vi "Write File ini.vi"(8 "error in (no error)":errorcluster, 11 "ini Path":path) -> (0 "error out":errorcluster)   [LabVIEW 2015, in "Telegram Library.lvlib"]
doc: "Created IvanLis by LabVIEW Portal\nProfile: http://labviewportal.org/memberlist.php?mode=viewprofile&u=987\neMail: IvanLisanov@gMail.com\nTelegram: https://t.me/IvanLis"
uses:
  Telegram Library.lvlib
  <vilib>/Utility/config.llb/Write Key (String).vi
  <vilib>/Utility/config.llb/Write Key (Boolean).vi
  <vilib>/Utility/config.llb/Write Key (I32).vi
  <vilib>/Utility/config.llb/NI_LVConfig.lvlib
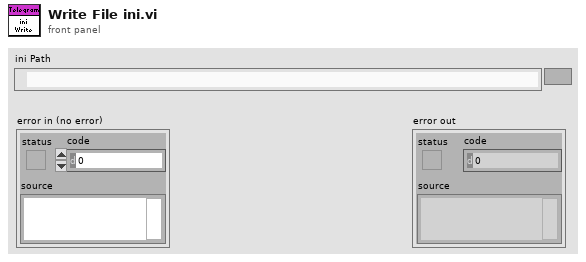
[diagram p1: front panel]
types:
  T1 = typedef "NI_LVConfig.lvlib/Config Data RefNum.ctl" = refnum<k1>
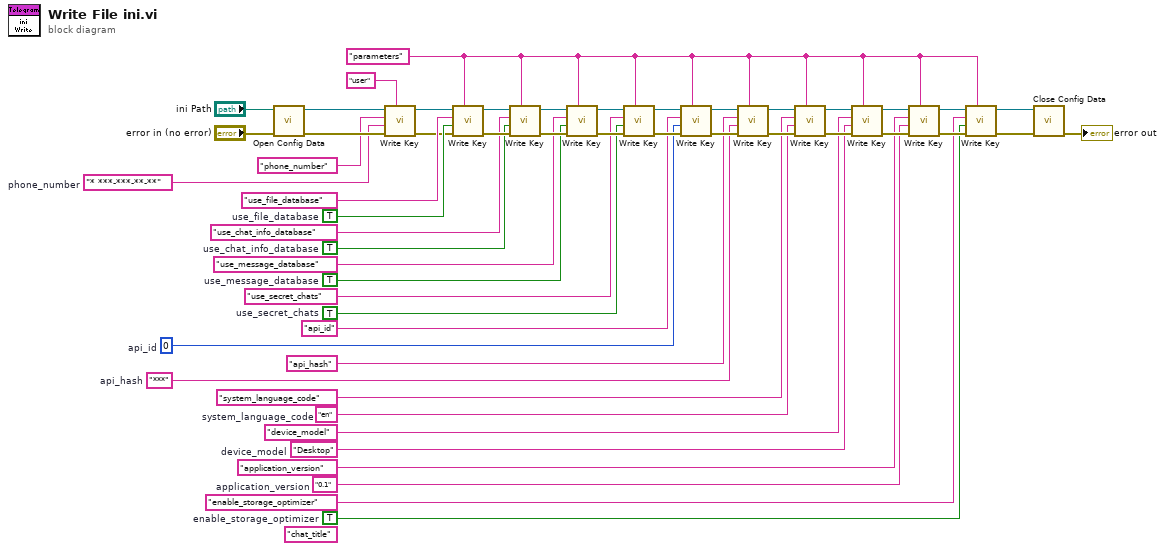
[diagram p0: block diagram]
diagram:
  w6 = TRUE  # enable_storage_optimizer
  w8 = "0.1"  # application_version
  w10 = "Desktop"  # device_model
  w12 = "en"  # system_language_code
  w14 = "***"  # api_hash
  w16 = 0  # api_id
  w18 = TRUE  # use_secret_chats
  w20 = TRUE  # use_message_database
  w22 = TRUE  # use_chat_info_database
  w23 = TRUE  # use_file_database
  w25 = "parameters"
  (unwired) "chat_title"
  w47 = "* ***-***-**-**"  # phone_number
  n1 = call <vilib>:"Open Config Data.vi"("error in (no error)"="error in (no error)", "configuration file path"="ini Path") -> ("error out"=w48:errorcluster, "refnum"=w49:T1)  [unwired: 7 in, 1 out]
  n2 = call-poly <vilib>:"Write Key.vi"("section"="user", "error in (no error)"=w48, "value"=w47, "key"="phone_number", "refnum"=w49) -> ("error out"=w3:errorcluster, "refnum out"=w4:T1)  [unwired: 4 in, 1 out]
  n3 = call-poly <vilib>:"Write Key.vi"("section"=w25, "error in (no error)"=w3, "value"=w23, "key"="use_file_database", "refnum"=w4) -> ("error out"=w30:errorcluster, "refnum out"=w41:T1)  [unwired: 4 in, 1 out]
  n4 = call-poly <vilib>:"Write Key.vi"("section"=w25, "error in (no error)"=w30, "value"=w22, "key"="use_chat_info_database", "refnum"=w41) -> ("error out"=w29:errorcluster, "refnum out"=w40:T1)  [unwired: 4 in, 1 out]
  n5 = call-poly <vilib>:"Write Key.vi"("section"=w25, "error in (no error)"=w29, "value"=w20, "key"="use_message_database", "refnum"=w40) -> ("error out"=w28:errorcluster, "refnum out"=w39:T1)  [unwired: 4 in, 1 out]
  n6 = call-poly <vilib>:"Write Key.vi"("section"=w25, "error in (no error)"=w28, "value"=w18, "key"="use_secret_chats", "refnum"=w39) -> ("error out"=w27:errorcluster, "refnum out"=w38:T1)  [unwired: 4 in, 1 out]
  n7 = call-poly <vilib>:"Write Key.vi"("section"=w25, "error in (no error)"=w27, "value"=w16, "key"="api_id", "refnum"=w38) -> ("error out"=w26:errorcluster, "refnum out"=w37:T1)  [unwired: 4 in, 1 out]
  n8 = call-poly <vilib>:"Write Key.vi"("section"=w25, "error in (no error)"=w26, "value"=w14, "key"="api_hash", "refnum"=w37) -> ("error out"=w43:errorcluster, "refnum out"=w42:T1)  [unwired: 4 in, 1 out]
  n9 = call-poly <vilib>:"Write Key.vi"("section"=w25, "error in (no error)"=w43, "value"=w12, "key"="system_language_code", "refnum"=w42) -> ("error out"=w33:errorcluster, "refnum out"=w36:T1)  [unwired: 4 in, 1 out]
  n10 = call-poly <vilib>:"Write Key.vi"("section"=w25, "error in (no error)"=w33, "value"=w10, "key"="device_model", "refnum"=w36) -> ("error out"=w32:errorcluster, "refnum out"=w35:T1)  [unwired: 4 in, 1 out]
  n11 = call-poly <vilib>:"Write Key.vi"("section"=w25, "error in (no error)"=w32, "value"=w8, "key"="application_version", "refnum"=w35) -> ("error out"=w31:errorcluster, "refnum out"=w34:T1)  [unwired: 4 in, 1 out]
  n12 = call-poly <vilib>:"Write Key.vi"("section"=w25, "error in (no error)"=w31, "value"=w6, "key"="enable_storage_optimizer", "refnum"=w34) -> ("error out"=w1:errorcluster, "refnum out"=w2:T1)  [unwired: 4 in, 1 out]
  n13 = call <vilib>:"Close Config Data.vi"("error in (no error)"=w1, "refnum"=w2) -> ("error out"=→"error out":errorcluster)  [unwired: 8 in, 1 out]
